vi "exitMaintenance.vi"(8 "error in (no error)":errorcluster, 10 "Parameters":T1, 11 "Context in":refnum<class "Context.lvclass">) -> (0 "error out":errorcluster, 3 "Context out":refnum<class "Context.lvclass">)   [LabVIEW 2016, in "Context.lvclass"]
uses:
  Context.lvclass
  DataTypes/Topics/CommandExitMaintenance.ctl
  DataTypes/Topics/Parts/CommandId.ctl
  Context.lvclass/Context.ctl
  States/State/State.lvclass
  Model/Model.lvclass
  DataTypes/Topics/M1M3SupportTopics.lvlib
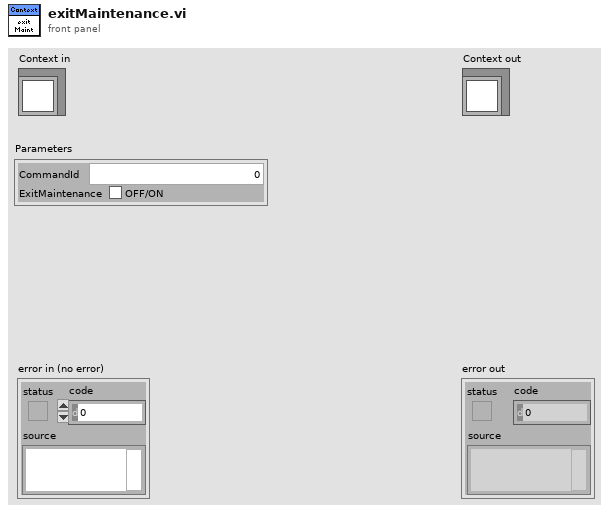
[diagram p1: front panel]
types:
  T1 = typedef "M1M3SupportTopics.lvlib/CommandExitMaintenance.ctl" = cluster{"CommandId":T2, "ExitMaintenance":bool}
  T2 = typedef "M1M3SupportTopics.lvlib/CommandId.ctl" = i32
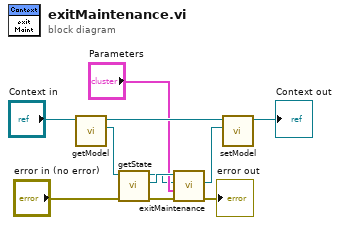
[diagram p0: block diagram]
diagram:
  n1 = call "getModel.vi"("Context in"="Context in") -> ("Model"=w10:refnum<class "Model.lvclass">, "Context out"=w9:refnum<class "Context.lvclass">)  [unwired: 9 in]
  n2 = call "getState.vi"("error in (no error)"="error in (no error)", "Model in"=w10) -> ("error out"=w5:errorcluster, "State out"=w11:refnum<class "State.lvclass">, "Model out"=w2:refnum<class "Model.lvclass">)  [unwired: 7 in]
  n3 = call-dynamic "exitMaintenance.vi"("error in (no error)"=w5, "Parameters"="Parameters", "Model in"=w2, "State in"=w11) -> ("error out"=→"error out":errorcluster, "Model out"=w1:refnum<class "Model.lvclass">)  [unwired: 5 in, 1 out]
  n4 = call "setModel.vi"("Model"=w1, "Context in"=w9) -> ("Context out"=→"Context out":refnum<class "Context.lvclass">)  [unwired: 9 in]
